vi "Periodic Tasks.vi"(8 "error in":errorcluster) -> ()   [LabVIEW 2016]
doc: "This VI runs in parallel to other tasks. It can contain as many user-defined periodic loops as you need. These can carry out PID or other sorts of timed response."
uses:
  Robot Global Data.vi
  <vilib>/Rock Robotics/Network Tables/NT Write Number.vi
panel:
  out "Right Encoder":dbl format="%#_13g"
  out "Left Encoder":dbl format="%#_13g"
  out "angle":dbl format="%#_13g"
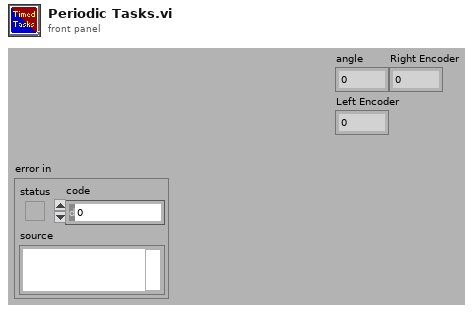
[diagram p1: front panel]
types:
  T1 = typedef "WPI_GyroDevRef.ctl" = cluster{"DevStatus":errorcluster, "Analog Channel":T2, "Offset":dbl, "Gain (VoltsPerDegree/Second)":dbl, "Gyro Type":enum16{"Analog", "XRS450"}, "Handle":i32, "SPI Bus":T3, "Device Found":bool, "Sample Rate":dbl, "Calibrate On Open":bool}
  T2 = typedef "FPGA_AIChannel.ctl" = enum8{"AI 0", "AI 1", "AI 2", "AI 3", "AI MXP 0", "AI MXP 1", "AI MXP 2", "AI MXP 3", "Invalid"}
  T3 = typedef "spi_bus.ctl" = enum16{"SPI On-Board, CS0", "SPI On-Board, CS1", "SPI On-Board, CS2", "SPI On-Board, CS3", "SPI MXP", "Invalid"}
  T4 = typedef "WPI_EncoderDevRef.ctl" = cluster{"DevStatus":errorcluster, "EncoderIndex":T5, "CounterIndex":T6, "DistancePerCount":dbl, "Decoding Type":T7}
  T5 = typedef "FPGA_EncoderIdx.ctl" = enum8{"Enc 0", "Enc 1", "Enc 2", "Enc 3", "Enc 4", "Enc 5", "Enc 6", "Enc 7", "Invalid"}
  T6 = typedef "FPGA_CounterCtrSystemIndex.ctl" = enum8{"Ctr 0", "Ctr 1", "Ctr 2", "Ctr 3", "Ctr 4", "Ctr 5", "Ctr 6", "Ctr 7", "Invalid"}
  T7 = typedef "WPI_EncoderType.ctl" = enum16{"1x", "2x", "4x"}
  T8 = typedef "WPI_AnalogChannelDevRef.ctl" = cluster{"DevStatus":errorcluster, "Analog Channel":T2}
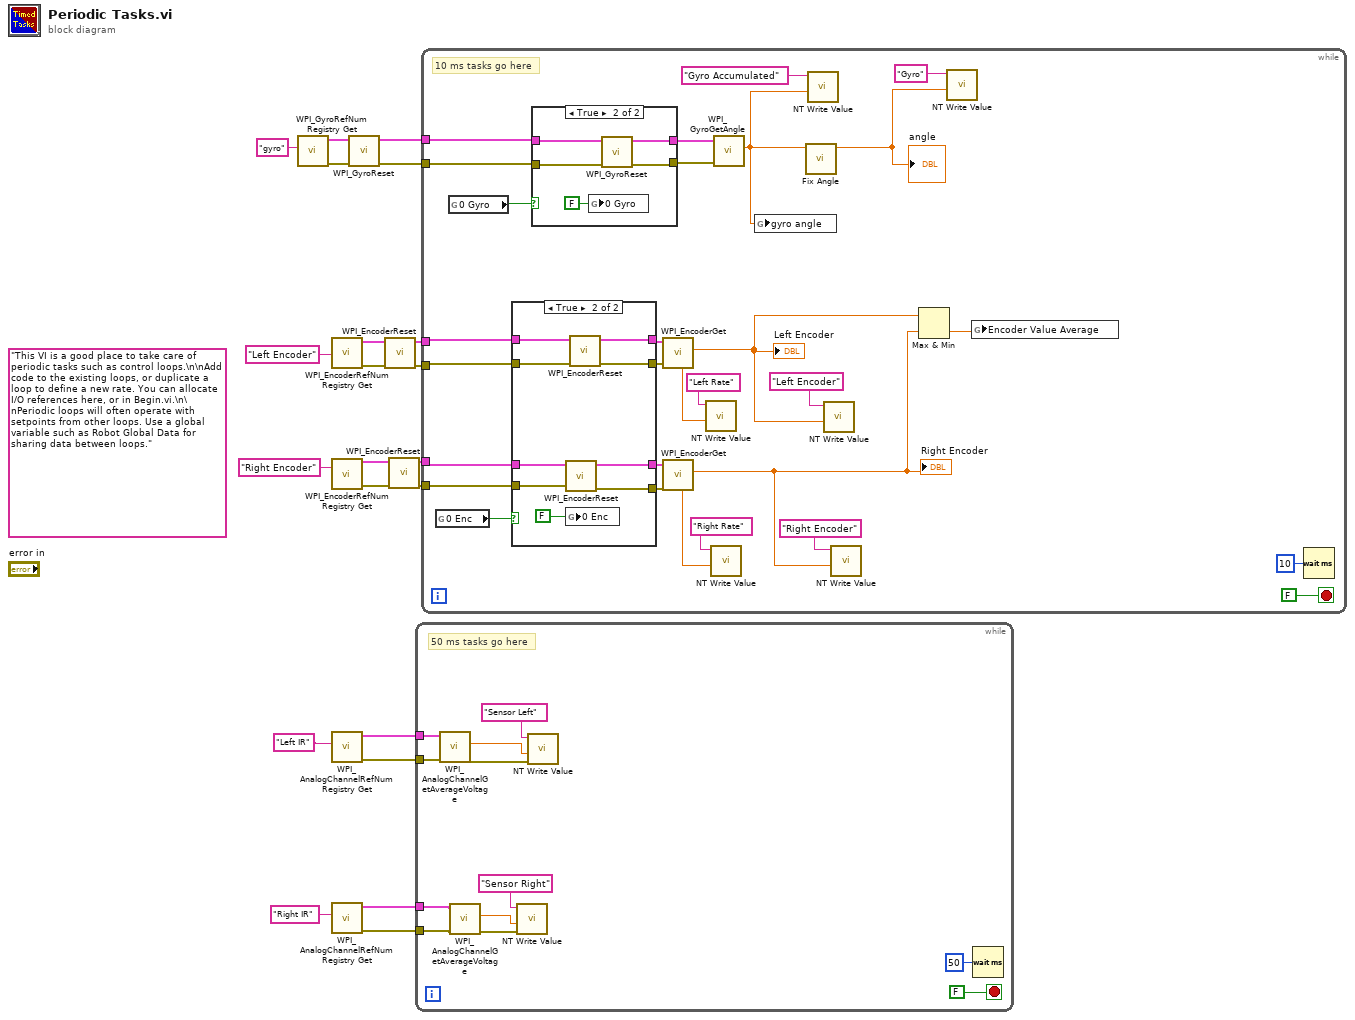
[diagram p0: block diagram]
diagram:
  (unwired) "This VI is a good place to take care of periodic tasks such as control loops.\n\nAdd code to the existing loops, or duplicate a loop to define a new rate. You can allocate I/O references here, or in Begin.vi.\n\nPeriodic loops will often operate with setpoints from other loops. Use a global variable such as Robot Global Data for sharing data between loops."
  n1 = call <vilib>:"WPI_GyroRefNum Registry Get.vi"("refnum name"="gyro") -> ("error out"=w20:errorcluster, "GyroDevRef"=w19:T1)  [unwired: 9 in]
  n2 = call <vilib>:"WPI_EncoderRefNum Registry Get.vi"("refnum name"="Left Encoder") -> ("error out"=w14:errorcluster, "EncoderDevRef"=w13:T4)  [unwired: 9 in]
  n3 = call <vilib>:"WPI_EncoderRefNum Registry Get.vi"("refnum name"="Right Encoder") -> ("error out"=w11:errorcluster, "EncoderDevRef"=w12:T4)  [unwired: 9 in]
  n4 = call <vilib>:"WPI_AnalogChannelRefNum Registry Get.vi"("refnum name"="Left IR") -> ("error out"=w4:errorcluster, "AIDeviceRef"=w5:T8)  [unwired: 9 in]
  n5 = call <vilib>:"WPI_AnalogChannelRefNum Registry Get.vi"("refnum name"="Right IR") -> ("error out"=w1:errorcluster, "AIDeviceRef"=w2:T8)  [unwired: 9 in]
  n6 = call <vilib>:"WPI_GyroReset.vi"("error in"=w20, "GyroDevRef"=w19) -> ("error out"=w17:errorcluster, "GyroDevRef"=w18:T1)  [unwired: 8 in]
  n7 = call <vilib>:"WPI_EncoderReset.vi"("error in (no error)"=w14, "EncoderDevRef"=w13) -> ("error out"=w9:errorcluster, "EncoderDevRef"=w10:T4)  [unwired: 8 in]
  n8 = call <vilib>:"WPI_EncoderReset.vi"("error in (no error)"=w11, "EncoderDevRef"=w12) -> ("error out"=w7:errorcluster, "EncoderDevRef"=w8:T4)  [unwired: 8 in]
  n9 = while {
    tunnel: w5 -> [w31]
    tunnel: w4 -> [w30]
    tunnel: w2 -> [w26]
    tunnel: w1 -> [w25]
    stop <- FALSE stop-if-true
    # "50 ms tasks go here"
    n10 = call <vilib>:"WPI_AnalogChannelGetAverageVoltage.vi"("error in (no error)"=w30, "AIDeviceRef"=w31) -> ("error out"=w28:errorcluster, "Voltage"=w29:dbl)  [unwired: 7 in, 1 out]
    n11 = call <vilib>:"WPI_AnalogChannelGetAverageVoltage.vi"("error in (no error)"=w25, "AIDeviceRef"=w26) -> ("error out"=w24:errorcluster, "Voltage"=w23:dbl)  [unwired: 7 in, 1 out]
    n12 = call-poly <vilib>:"NT Write Value.vi"("error in"=w24, "Numeric"=w23, "Name"="Sensor Right") -> ()  [unwired: 8 in, 1 out]
    n13 = call-poly <vilib>:"NT Write Value.vi"("error in"=w28, "Numeric"=w29, "Name"="Sensor Left") -> ()  [unwired: 8 in, 1 out]
    n14 = Wait (ms)(milliseconds to wait=u32 50) -> ()  [unwired: 1 out]
  }
  n15 = while {
    tunnel: w18 -> [w56]
    tunnel: w17 -> [w54]
    tunnel: w10 -> [w53]
    tunnel: w9 -> [w51]
    tunnel: w8 -> [w48]
    tunnel: w7 -> [w47]
    stop <- FALSE stop-if-true
    # "10 ms tasks go here"
    n16 = global read "Robot Global Data.vi" "0 Enc"() -> (w46:bool)
    n17 = global read "Robot Global Data.vi" "0 Gyro"() -> (w55:bool)
    n18 = case shown="True" w46 {
      tunnel: w53 -> [w66 w74]
      tunnel: [w66 w73] -> w45
      tunnel: [w65 w72] -> w52
      tunnel: w51 -> [w65 w71]
      tunnel: [w64 w70] -> w50
      tunnel: [w63 w69] -> w49
      tunnel: w48 -> [w64 w68]
      tunnel: w47 -> [w63 w67]
      frame False {
      }
      frame True {
        n19 = call <vilib>:"WPI_EncoderReset.vi"("error in (no error)"=w67, "EncoderDevRef"=w68) -> ("error out"=w69:errorcluster, "EncoderDevRef"=w70:T4)  [unwired: 8 in]
        n20 = global write "Robot Global Data.vi" "0 Enc"(FALSE ("0 Gyro")) -> ()
        n21 = call <vilib>:"WPI_EncoderReset.vi"("error in (no error)"=w71, "EncoderDevRef"=w74) -> ("error out"=w72:errorcluster, "EncoderDevRef"=w73:T4)  [unwired: 8 in]
      }
    }
    n22 = case shown="True" w55 {
      tunnel: w56 -> [w77 w82]
      tunnel: [w76 w81] -> w58
      tunnel: [w77 w80] -> w57
      tunnel: w54 -> [w76 w78]
      frame False {
      }
      frame True {
        n23 = global write "Robot Global Data.vi" "0 Gyro"(FALSE ("0 Gyro")) -> ()
        n24 = call <vilib>:"WPI_GyroReset.vi"("error in"=w78, "GyroDevRef"=w82) -> ("error out"=w81:errorcluster, "GyroDevRef"=w80:T1)  [unwired: 8 in]
      }
    }
    n25 = call <vilib>:"WPI_EncoderGet.vi"("error in (no error)"=w52, "EncoderDevRef"=w45) -> ("Distance"=w44:dbl, "Rate"=w42:dbl)  [unwired: 4 in, 4 out]
    "Left Encoder" <- w44
    n26 = call <vilib>:"WPI_EncoderGet.vi"("error in (no error)"=w49, "EncoderDevRef"=w50) -> ("Distance"=w34:dbl, "Rate"=w40:dbl)  [unwired: 4 in, 4 out]
    "Right Encoder" <- w34
    n27 = call-poly <vilib>:"NT Write Value.vi"("Numeric"=w42, "Name"="Left Rate") -> ()  [unwired: 9 in, 1 out]
    n28 = call-poly <vilib>:"NT Write Value.vi"("Numeric"=w40, "Name"="Right Rate") -> ()  [unwired: 9 in, 1 out]
    n29 = call <vilib>:"WPI_GyroGetAngle.vi"("error in"=w58, "GyroDevRef"=w57) -> ("Angle"=w37:dbl)  [unwired: 5 in, 4 out]
    n30 = global write "Robot Global Data.vi" "gyro angle"(w37) -> ()
    n31 = call "Fix Angle.vi"("Angle In"=w37) -> ("Angle Out"=w35:dbl)  [unwired: 10 in]
    "angle" <- w35
    n32 = call-poly <vilib>:"NT Write Value.vi"("Numeric"=w37, "Name"="Gyro Accumulated") -> ()  [unwired: 9 in, 1 out]
    n33 = call-poly <vilib>:"NT Write Value.vi"("Numeric"=w44, "Name"="Left Encoder") -> ()  [unwired: 9 in, 1 out]
    n34 = call-poly <vilib>:"NT Write Value.vi"("Numeric"=w34, "Name"="Right Encoder") -> ()  [unwired: 9 in, 1 out]
    n35 = Max & Min(x=w44, y=w34) -> (min(x,y)=w43:dbl)  [unwired: 1 out]
    n36 = call-poly <vilib>:"NT Write Value.vi"("Numeric"=w35, "Name"="Gyro") -> ()  [unwired: 9 in, 1 out]
    n37 = global write "Robot Global Data.vi" "Encoder Value Average"(w43) -> ()
    n38 = Wait (ms)(milliseconds to wait=u32 10) -> ()  [unwired: 1 out]
  }
